vi "Subvi pixel clock improv unfinished.vi"   [LabVIEW 2017]
uses:
  <vilib>/Platform/TimedLoop/XDataNode/timing_clust.ctl
  <vilib>/Platform/TimedLoop/XDataNode/nitl_modes.ctl
  <vilib>/Platform/TimedLoop/XDataNode/wakeup.ctl
  <vilib>/rvi/Emulation/niFpgaSctlEmulationGetInTimedLoop.vi
  <vilib>/rvi/Emulation/niFpgaEmulationReportErrorSimple.vi
  <vilib>/rvi/Emulation/niFpgaGetClockAttributes.vi
  <vilib>/rvi/Emulation/niFpgaCriticalErrorInLSC.vi
  <vilib>/rvi/Emulation/niFpgaProcessEmulError.vi
  <vilib>/rvi/eio/common/nirviEmuTemplateMethod_errors.vi
  GV N pixel clock per line.vi
  <vilib>/rvi/Memory/Memory_Emulation/nirvimemoryFastEmulation.vi
  <vilib>/rvi/Memory/Memory_Emulation/nirvimemoryEmulation.vi
  <vilib>/rvi/Emulation/niFpgaEmulationIsFPGAContextNoSignature.vi
  <vilib>/rvi/DataTransferAndStorage/Container/Common/niFpgaContainerGetUniqueNameForEmu.vi
  <vilib>/rvi/errors/nirviReportUnexpectedCaseInternalError (U32).vi
  <vilib>/Platform/TimedLoop/XDataNode/XDataNode.xnode
  <vilib>/eio/EIONode/EIONode.xnode
  <vilib>/rvi/DataTransferAndStorage/Container/XNode/niFpgaContainer.xnode
  <vilib>/Platform/TimedLoop/XDataNode/XDNodeRunTimeDep.lvlib
  GV pixel clock.vi
  GV line clock change.vi
types:
  T1 = typedef "XDNodeRunTimeDep.lvlib/timing_clust.ctl" = cluster{"Expected End [f-1]":u64, "Actual End [f-1]":u64, "Finished Late? [f-1]":bool, "Expected End [i-1]":u64, "Actual End [i-1]":u64, "Finished Late? [i-1]":bool, "Expected Start [i]":u64, "Actual Start [i]":u64, "Expected Start [f]":u64, "Actual Start [f]":u64, "Source Name":string, "Structure Name":string, "Period":i64, "Deadline":i64, "Offset":i64, "Start":i64, "Priority":i32, "Timeout":i32, "Mode":T2, "Wakeup Reason":T3, "Error":errorcluster, "Source Type":string, "Secondary Source Type":string, "Global End Time":u64, "Global Start Time":u64, "Frame Duration":u64, "Iteration Duration":u64, "Assigned CPU":i32, "I/O Scan Engine Mode":u32}
  T2 = typedef "XDNodeRunTimeDep.lvlib/nitl_modes.ctl" = enum32{"No Change", "Process missed periods, maintain original phase", "Discard missed periods, maintain original phase", "Process missed periods, ignore original phase", "Discard missed periods, ignore original phase"}
  T3 = typedef "XDNodeRunTimeDep.lvlib/wakeup.ctl" = enum32{"Normal", "Aborted", "Asynchronous wakeup", "Timing source error", "Timed loop error", "Timeout"}
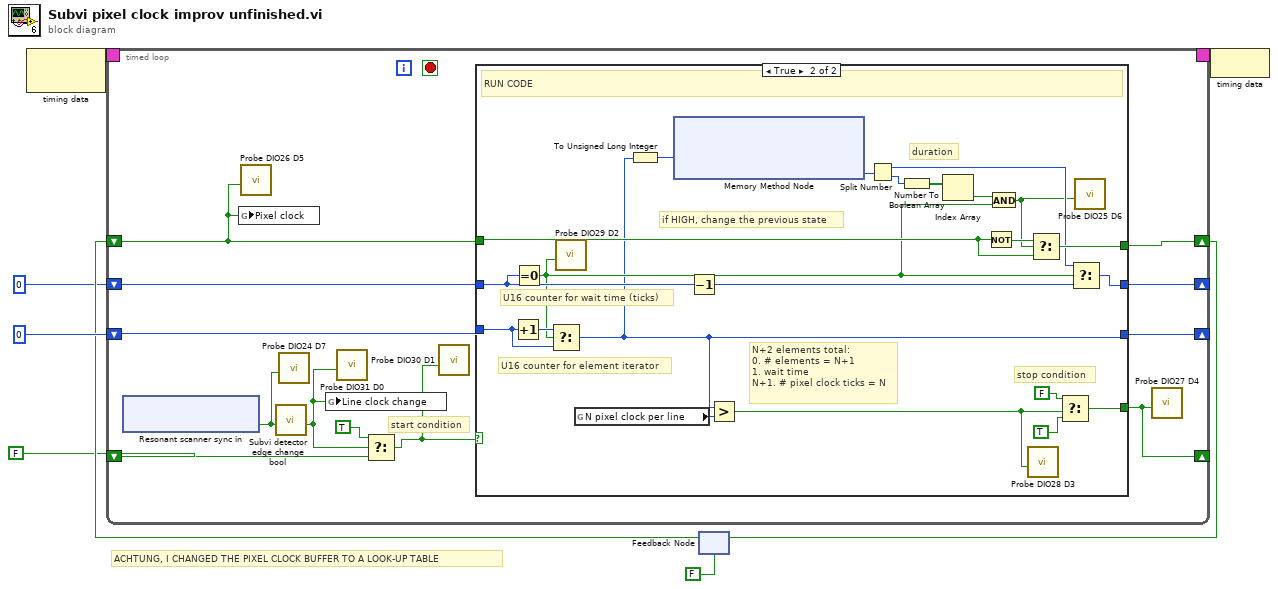
[diagram p0: block diagram]
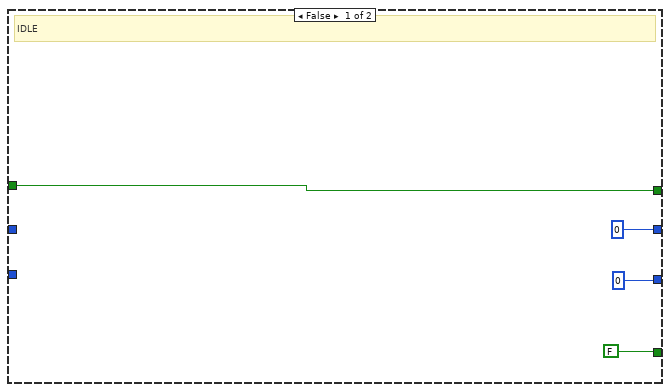
[diagram p2: hidden frame]
diagram:
  # "ACHTUNG, I CHANGED THE PIXEL CLOCK BUFFER TO A LOOK-UP TABLE"
  n1 = node-c288() -> (w8:T1)  [unwired: 1 in]
  n2 = feedback #1(FALSE) -> (w4:bool)
  n3 = timed-loop {
    timing: w8 -> [_]
    timing-out: [_] -> w7
    shift-right: [w18] -> _
    shift-left: u16 0 -> [w19]
    shift-right: [w12] -> _
    shift-left: FALSE -> [w16]
    shift-right: [w17] -> w3
    shift-left: w4 -> [w11]
    shift-right: [w14] -> _
    shift-left: u16 0 -> [w15]
    stop <- _ stop-if-true
    # "start condition"
    n4 = xnode "Resonant scanner sync in"() -> ("Connector0/DIO0"=w10:bool)  [unwired: 1 in, 1 out]
    n5 = global write "GV pixel clock.vi" "Pixel clock"(w11) -> ()
    n6 = call "Probe DIO26 D5.vi"("D5"=w11) -> ()  [unwired: 11 in]
    n7 = call "Subvi detector edge change bool.vi"("Input"=w10) -> ("Output"=w9:bool)  [unwired: 8 in]
    n8 = call "Probe DIO24 D7.vi"("D7"=w10) -> ()  [unwired: 11 in]
    n9 = global write "GV line clock change.vi" "Line clock change"(w9) -> ()
    n10 = call "Probe DIO31 D0.vi"("D0"=w9) -> ()  [unwired: 11 in]
    n11 = Select(t=TRUE, s=w9, f=w16) -> (s? t:f=w13:bool)
    n12 = call "Probe DIO30 D1.vi"("D1"=w13) -> ()  [unwired: 11 in]
    n13 = case shown="True" w13 {
      tunnel: [FALSE w45] -> w12
      tunnel: w19 -> [_ w35]
      tunnel: [u16 0 w38] -> w18
      tunnel: [w24 w39] -> w17
      tunnel: w11 -> [w24 w36]
      tunnel: w15 -> [_ w32]
      tunnel: [u16 0 w31] -> w14
      frame False {
        # "IDLE"
      }
      frame True {
        # "U16 counter for wait time (ticks)"
        # "if HIGH, change the previous state"
        # "N+2 elements total:\n0. # elements = N+1\n1. wait time \nN+1. # pixel clock ticks = N"
        # "duration"
        # "U16 counter for element iterator"
        # "stop condition"
        # "RUN CODE"
        n14 = Increment(x=w32) -> (x+1=w43:u16)
        n15 = Equal To 0?(x=w35) -> (x = 0?=w33:bool)
        n16 = Select(t=w43, s=w33, f=w32) -> (s? t:f=w31:u16)
        n17 = call "Probe DIO29 D2.vi"("D2"=w33) -> ()  [unwired: 11 in]
        n18 = global read "GV N pixel clock per line.vi" "N pixel clock per line"() -> (w25:u16)
        n19 = To Unsigned Long Integer(number=w31) -> (unsigned 32bit integer=w27:u32)
        n20 = xnode ("Memory Method Node")("Address"=w27) -> ("Data"=w26:u32)  [unwired: 1 in, 1 out]
        n21 = Decrement(x=w35) -> (x-1=w29:u16)
        n22 = Greater?(x=w31, y=w25) -> (0:w30:bool)
        n23 = Split Number(x=w26) -> (hi(x)=w37:u16, lo(x)=w41:u16)
        n24 = Number To Boolean Array(number=w41) -> (Boolean array=w42:bool[])
        n25 = Index Array(array=w42) -> (element=w34:bool)  [unwired: 1 in]
        n26 = Not(x=w36) -> (.not. x?=w40:bool)
        n27 = And(x=w34, y=w33) -> (x .and. y?=w28:bool)
        n28 = call "Probe DIO28 D3.vi"("D3"=w30) -> ()  [unwired: 11 in]
        n29 = Select(t=w40, s=w28, f=w36) -> (s? t:f=w39:bool)
        n30 = Select(t=FALSE, s=w30, f=TRUE) -> (s? t:f=w45:bool)
        n31 = Select(t=w37, s=w33, f=w29) -> (s? t:f=w38:u16)
        n32 = call "Probe DIO25 D6.vi"("D6"=w28) -> ()  [unwired: 11 in]
      }
    }
    n33 = call "Probe DIO27 D4.vi"("D4"=w12) -> ()  [unwired: 11 in]
  }
  n34 = feedback-in #1(w3) -> ()
  n35 = node-c288(w7) -> ()
